vi "PXI-Write AO Buffers E.vi"(0 "AO Tasks":T2[](array[typedef]), 3 "BufferSize":i32, 7 "AO Waveforms":dbl[][](array[numeric]), 9 "Ramping":T1={"Ramp up?"=FALSE, "Ramp down?"=FALSE, "Ramp duration (msecs)"=0.005, "Ramp type"=enum."Cos2"}, 11 "error in (no error)":errorcluster, 12 "Force write":bool, 13 "zero output":bool) -> (4 "AO Tasks out":T2[](array[typedef]), 15 "error out":errorcluster)   [LabVIEW 2020]
uses:
  Type Defs/Task Struct.ctl
  Type Defs/Ramping Params.ctl
  <vilib>/DAQmx/write.llb/DAQmx Write (Analog 2D DBL NChan NSamp).vi
  <vilib>/DAQmx/write.llb/DAQmx Write (Analog 1D DBL 1Chan NSamp).vi
  PXI Globals.vi
  Utility VIs/Array Manipulation VIs/Array-Dimensions (2D).vi
  <vilib>/DAQmx/miscellaneous.llb/DAQmx Fill In Error Info.vi
panel:
  out "Waveform Graph":dbl[][](graph)
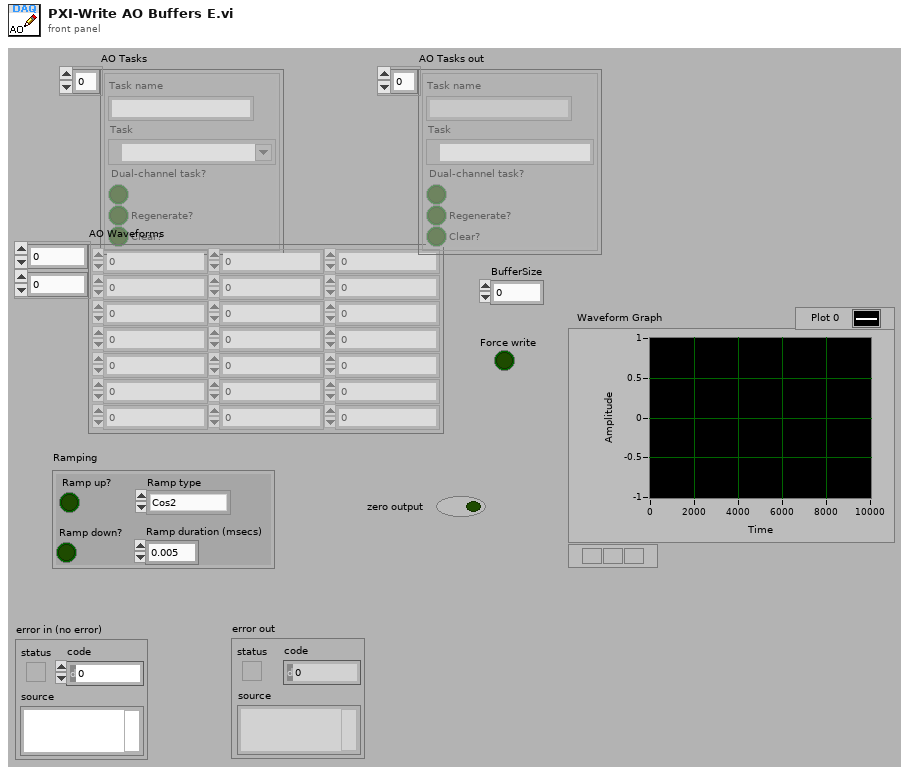
[diagram p1: front panel]
types:
  T1 = typedef "Ramping Params.ctl" = cluster{"Ramp up?":bool, "Ramp down?":bool, "Ramp duration (msecs)":dbl, "Ramp type":enum16{"Linear", "Cos2"}}
  T2 = typedef "Task Struct.ctl" = cluster{"Task name":string, "Task":refnum<k21>, "Dual-channel task?":bool, "Regenerate?":bool, "Clear?":bool}
  T3 = enum16{"Init", "Write", "Read", "Latch setup", "Compute comp."}
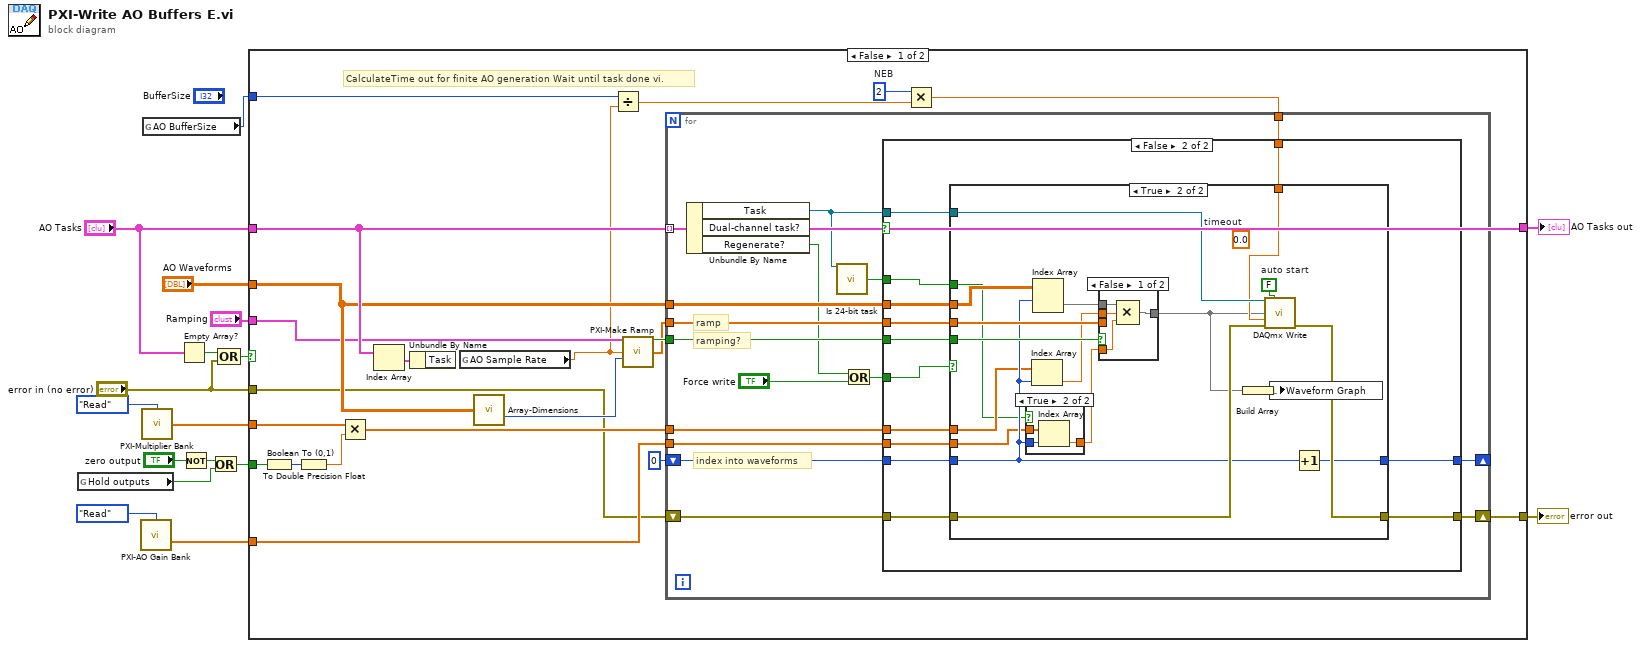
[diagram p0: block diagram]
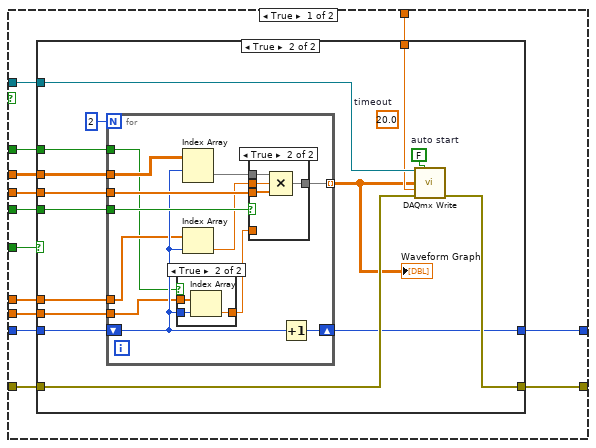
[diagram p2: hidden frame]
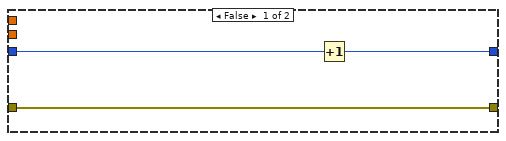
[diagram p3: hidden frame]
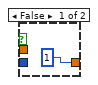
[diagram p4: hidden frame]
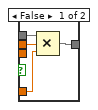
[diagram p5: hidden frame]
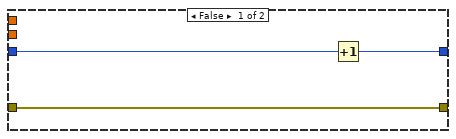
[diagram p6: hidden frame]
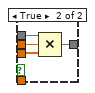
[diagram p7: hidden frame]
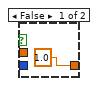
[diagram p8: hidden frame]
diagram:
  n1 = global read "PXI Globals.vi" "Hold outputs"() -> (w1:bool)
  n2 = call "PXI-AO Gain Bank.vi"("Action"=T3."Read") -> ("Gain Compensation Factors"=w10:dbl[])  [unwired: 9 in, 5 out]
  n3 = call "PXI-Multiplier Bank.vi"("Action"=enum16{"Init", "Write", "Read"}."Read") -> ("Multipliers out"=w12:dbl[])  [unwired: 12 in, 2 out]
  n4 = global read "PXI Globals.vi" "AO BufferSize"() -> (w6:i32)
  n5 = Empty Array?(array="AO Tasks") -> (empty?=w4:bool)
  n6 = Not(x="zero output") -> (.not. x?=w7:bool)
  n7 = Or(x=w7, y=w1) -> (x .or. y?=w2:bool)
  n8 = Compound Arithmetic op=OR(w4, "error in (no error)") -> (w16:bool)
  n9 = case shown="False" w16 {
    tunnel: [w38 w158] -> w17
    tunnel: "error in (no error)" -> [w18 w158]
    tunnel: "AO Tasks" -> [w32 w157]
    tunnel: [w32 w157] -> w15
    tunnel: w12 -> [w28 _]
    tunnel: w10 -> [w27 _]
    tunnel: "Ramping" -> [w20 _]
    tunnel: "AO Waveforms" -> [w26 _]
    tunnel: w6 -> [w25 _]
    tunnel: w2 -> [w24 _]
    frame False {
      w29 = 2  # NEB
      # "CalculateTime out for finite AO generation Wait until task done vi."
      n10 = Boolean To (0,1)(Boolean=w24) -> (0, 1=w23:i16)
      n11 = To Double Precision Float(number=w23) -> (double precision float=w21:dbl)
      n12 = Multiply(x=w28, y=w21) -> (x*y=w22:dbl[])
      n13 = Index Array(array=w32) -> (element=w36:T2)  [unwired: 1 in]
      n14 = Unbundle By Name(w36) -> ()  [unwired: 1 out]
      n15 = global read "PXI Globals.vi" "AO Sample Rate"() -> (w19:dbl)
      n16 = call-poly "Array-Dimensions.vi"("2D Array"=w26) -> ("# columns"=w35:i32)  [unwired: 13 in, 1 out]
      n17 = Divide(x=w25, y=w19) -> (x/y=w31:dbl)
      n18 = call "PXI-Make Ramp.vi"("Ramping"=w20, "Sampling rate (Hz)"=w19, "# samples"=w35) -> ("Ramping?"=w34:bool, "Ramp out"=w33:dbl[])  [unwired: 11 in]
      n19 = Multiply(x=w29, y=w31) -> (x*y=w30:dbl)
      n20 = for {
        tunnel: w32 -> [w44] mode=indexing
        shift-right: [w54] -> w38
        shift-left: w18 -> [w55]
        tunnel: w33 -> [w52]
        tunnel: w34 -> [w51]
        shift-right: [w47] -> _
        shift-left: 0 -> [w49]
        tunnel: w22 -> [w48]
        tunnel: w26 -> [w53]
        tunnel: w30 -> [w46]
        tunnel: w27 -> [w45]
        # "index into waveforms"
        # "ramping?"
        # "ramp"
        n21 = Unbundle By Name(w44) -> ("Task"=w43:refnum<k21>, "Dual-channel task?"=w50:bool, "Regenerate?"=w39:bool)
        n22 = call "Is 24-bit task.vi"("task"=w43) -> ("is 24bit?"=w42:bool)  [unwired: 9 in, 5 out]
        n23 = Or(x=w39, y="Force write") -> (x .or. y?=w41:bool)
        n24 = case shown="False" w50 {
          tunnel: w43 -> [w68 w123]
          tunnel: w55 -> [w67 w122]
          tunnel: [w66 w121] -> w54
          tunnel: w53 -> [w62 w117]
          tunnel: w52 -> [w65 w120]
          tunnel: w51 -> [w64 w119]
          tunnel: w49 -> [w61 w116]
          tunnel: [w60 w115] -> w47
          tunnel: w48 -> [w63 w118]
          tunnel: w41 -> [w59 w114]
          tunnel: w46 -> [w58 w113]
          tunnel: w45 -> [w57 w112]
          tunnel: w42 -> [w56 w111]
          frame True {
            n25 = case shown="True" w59 {
              tunnel: w68 -> [_ w86]
              tunnel: w67 -> [w71 w85]
              tunnel: [w71 w84] -> w66
              tunnel: w65 -> [_ w82]
              tunnel: w64 -> [_ w81]
              tunnel: w63 -> [_ w80]
              tunnel: w62 -> [_ w79]
              tunnel: w61 -> [w69 w77]
              tunnel: [w70 w76] -> w60
              tunnel: w58 -> [_ w75]
              tunnel: w57 -> [_ w74]
              tunnel: w56 -> [_ w73]
              frame False {
                n26 = Increment(x=w69) -> (x+1=w70:i32)
              }
              frame True {
                (unwired) 20.0  # timeout
                w83 = FALSE  # auto start
                n27 = for {
                  N: 2 -> [_]
                  tunnel: w82 -> [w94]
                  tunnel: w81 -> [w98]
                  tunnel: w80 -> [w91]
                  tunnel: w79 -> [w95]
                  tunnel: [w87] -> w72 mode=indexing
                  shift-right: [w96] -> w76
                  shift-left: w77 -> [w93]
                  tunnel: w74 -> [w90]
                  tunnel: w73 -> [w88]
                  n28 = case shown="True" w88 {
                    tunnel: w93 -> [_ w102]
                    tunnel: w90 -> [_ w101]
                    tunnel: [1 w100] -> w89
                    frame False {
                    }
                    frame True {
                      n29 = Index Array(array=w101, index=w102) -> (element=w100:dbl)
                    }
                  }
                  n30 = Index Array(array=w95, index (row)=w93) -> (element=w97:dbl[])  [unwired: 1 in]
                  n31 = Index Array(array=w91, index=w93) -> (element=w92:dbl)
                  n32 = case shown="True" w98 {
                    tunnel: w97 -> [w106 w110]
                    tunnel: [w105 w109] -> w87
                    tunnel: w94 -> [_ w108]
                    tunnel: w92 -> [w104 w107]
                    tunnel: w89 -> [w103 _]
                    frame False {
                      n33 = Compound Arithmetic op=MULTIPLY(w106, w104, w103) -> (w105:dbl[])
                    }
                    frame True {
                      n34 = Compound Arithmetic op=MULTIPLY(w110, w107, w108) -> (w109:dbl[])
                    }
                  }
                  n35 = Increment(x=w93) -> (x+1=w96:i32)
                }
                "Waveform Graph" <- w72
                n36 = call-poly <vilib>:"DAQmx Write.vi"("task/channels in"=w86, "auto start"=w83, "data"=w72, "timeout"=w75, "error in"=w85) -> ("error out"=w84:errorcluster)  [unwired: 8 in, 2 out]
              }
            }
          }
          frame False {
            n37 = case shown="True" w114 {
              tunnel: w123 -> [_ w144]
              tunnel: w122 -> [w126 w143]
              tunnel: [w126 w142] -> w121
              tunnel: w120 -> [_ w141]
              tunnel: w119 -> [_ w140]
              tunnel: w118 -> [_ w133]
              tunnel: w117 -> [_ w139]
              tunnel: w116 -> [w124 w134]
              tunnel: [w125 w138] -> w115
              tunnel: w113 -> [_ w129]
              tunnel: w112 -> [_ w131]
              tunnel: w111 -> [_ w130]
              frame False {
                n38 = Increment(x=w124) -> (x+1=w125:i32)
              }
              frame True {
                (unwired) 0.0  # timeout
                w137 = FALSE  # auto start
                n39 = case shown="True" w130 {
                  tunnel: [1.0 w156] -> w135
                  tunnel: w134 -> [_ w155]
                  tunnel: w131 -> [_ w154]
                  frame False {
                  }
                  frame True {
                    n40 = Index Array(array=w154, index=w155) -> (element=w156:dbl)
                  }
                }
                n41 = Index Array(array=w133, index=w134) -> (element=w132:dbl)
                n42 = Index Array(array=w139, index (row)=w134) -> (element=w136:dbl[])  [unwired: 1 in]
                n43 = case shown="False" w140 {
                  tunnel: w136 -> [w148 w152]
                  tunnel: [w147 w151] -> w127
                  tunnel: w141 -> [_ w150]
                  tunnel: w132 -> [w146 w149]
                  tunnel: w135 -> [w145 _]
                  frame False {
                    n44 = Compound Arithmetic op=MULTIPLY(w148, w146, w145) -> (w147:dbl[])
                  }
                  frame True {
                    n45 = Compound Arithmetic op=MULTIPLY(w152, w149, w150) -> (w151:dbl[])
                  }
                }
                n46 = Build Array(w127) -> (w128:dbl[][])
                n47 = call-poly <vilib>:"DAQmx Write.vi"("task/channels in"=w144, "auto start"=w137, "data"=w127, "timeout"=w129, "error in"=w143) -> ("error out"=w142:errorcluster)  [unwired: 8 in, 2 out]
                n48 = local write "Waveform Graph"(w128) -> ()
                n49 = Increment(x=w134) -> (x+1=w138:i32)
              }
            }
          }
        }
      }
    }
    frame True {
    }
  }
  "error out" <- w17
  "AO Tasks out" <- w15
